vi "TCP Chat Window Launcher.vi"() -> ()   [LabVIEW 2020]
uses:
  Protocols/TCP Strategy/TCP Stream Listener/TCP Stream Listener.lvclass
  C:/justACS/network-endpoints/4.0/Source/Protocols/TCP Strategy/TCP Stream/TCP Stream.lvclass
  C:/justACS/network-endpoints/4.0/Source/Abstract Classes/Message Stream/Message Stream.lvclass
  Chat Window/Chat Window.lvclass
  C:/Program Files (x86)/National Instruments/LabVIEW 2020/vi.lib/ActorFramework/Actor/Actor.lvclass
  Protocols/TCP Strategy/TCP Stream/TCP Stream.lvclass/TCP Stream.ctl
  Chat Window/Chat Window.lvclass/Chat Window.ctl
  Protocols/TCP Strategy/TCP Stream Initiator/TCP Stream Initiator.lvclass
  Protocols/TCP Strategy/TCP Stream/TCP Stream.lvclass
  <vilib>/ActorFramework/Actor/Actor.lvclass
panel:
  out "error out":errorcluster
  in  "local port":u16=2001
  in  "Remote Port":u16=2001
  in  "Remote Address":string="127.0.0.1"
  # "This VI launches two instances of a chat window actor.  The two chat windows launch nested endpoints, which connect via a TCP/IP message stream.\n\n1.  (Optional)  Specify the IP address for this machine, and the IP ports for the two enpoints.\n2.  Run this VI.\n3.  Stop the application by closing either chat window.\n\nAF_Debug_Trace is set to TRUE in this project, so you can follow the action with the Desktop Execution Trace Toolkit."
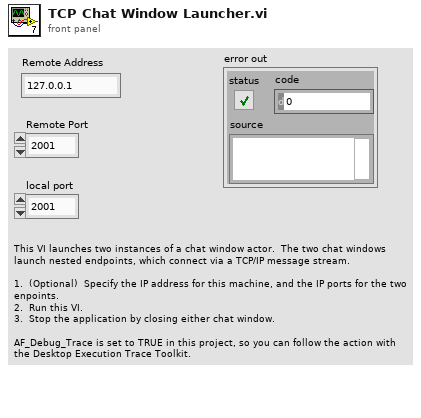
[diagram p1: front panel]
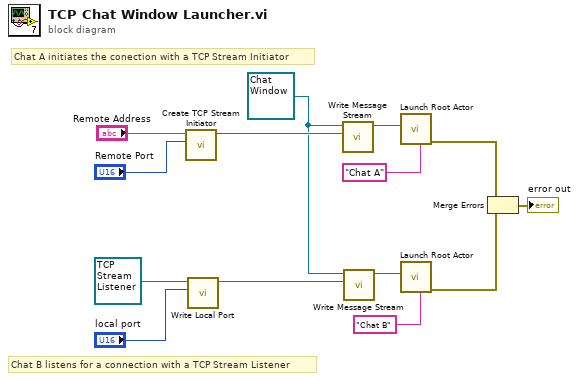
[diagram p0: block diagram]
diagram:
  w9 = refnum<class "Chat Window.lvclass"> refnum ("Chat Window in")
  # "Chat B listens for a connection with a TCP Stream Listener"
  # "Chat A initiates the conection with a TCP Stream Initiator"
  n1 = call "Create TCP Stream Initiator.vi"("Remote Port"="Remote Port", "Remote Address"="Remote Address") -> ("TCP Stream Initiator"=w10:refnum<class "TCP Stream Initiator.lvclass">)  [unwired: 9 in]
  n2 = call "Write Local Port.vi"("local port"="local port", "TCP Stream in"=refnum<class "TCP Stream Listener.lvclass"> refnum ("TCP Stream Listener.lvclass")) -> ("TCP Stream out"=w1:refnum<class "TCP Stream Listener.lvclass">)  [unwired: 9 in]
  n3 = call "Write Message Stream.vi"("Message Stream"=w10, "Chat Window in"=w9) -> ("Chat Window out"=w8:refnum<class "Chat Window.lvclass">)  [unwired: 9 in]
  n4 = call "Write Message Stream.vi"("Message Stream"=w1, "Chat Window in"=w9) -> ("Chat Window out"=w2:refnum<class "Chat Window.lvclass">)  [unwired: 9 in]
  n5 = call <vilib>:"Launch Root Actor.vi"("Debug Alias"="Chat A", "Actor"=w8) -> ("error out"=w5:errorcluster)  [unwired: 8 in, 1 out]
  n6 = call <vilib>:"Launch Root Actor.vi"("Debug Alias"="Chat B", "Actor"=w2) -> ("error out"=w4:errorcluster)  [unwired: 8 in, 1 out]
  n7 = Merge Errors(w5, w4) -> (→"error out":errorcluster)
